vi "EditOptions.vi"(8 "error in":errorcluster, 11 "node in":refnum<class "NISE_CEF_Node.lvclass">) -> (0 "error out":errorcluster, 1 "edit options":T1, 2 "subnodes class":T2, 3 "node out":refnum<class "NISE_CEF_Node.lvclass">)   [LabVIEW 2013, in "NISE_CEF_Node.lvclass"]
doc: "Contains the options for the Menu that will be displayed when doing right click on an item.\nThe sub nodes class configures which nodes can be added to this nodes\nAnd the edit options determine which options are available for the node.\nThis configuration is stored in this VI in case some dynamic configuration is required for the menu options or sub nodes."
uses:
  NISE_CEF_Node.lvclass
  SubNodeCluster.ctl
  NodeMenuOptions.ctl
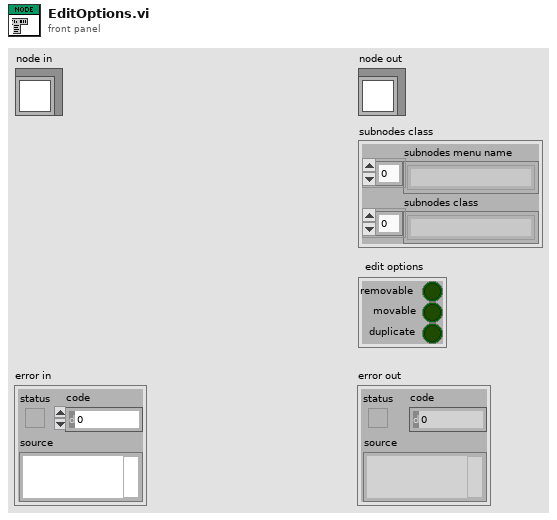
[diagram p1: front panel]
types:
  T1 = typedef "NISE_CEF_Node.lvclass/NodeMenuOptions.ctl" = cluster{"removable":bool, "movable":bool, "duplicate":bool}
  T2 = typedef "NISE_CEF_Node.lvclass/SubNodeCluster.ctl" = cluster{"subnodes menu name":string[], "subnodes class":string[]}
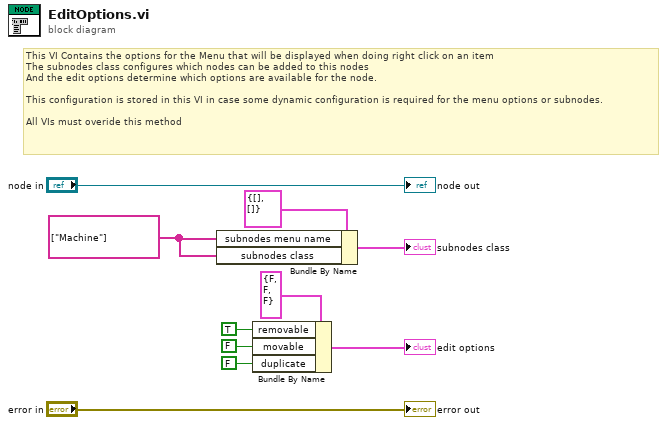
[diagram p0: block diagram]
diagram:
  w2 = string[] ["Machine"] ("subnodes class")
  # "This VI Contains the options for the Menu that will be displayed when doing right click on an item\nThe subnodes class configures which nodes can be added to this nodes\nAnd the edit options determine which options are available for the node.\n\nThis configuration is stored in this VI in case some dynamic configuration is required for the menu options or subnodes.\n\nAll VIs must overide this method"
  n1 = Bundle By Name(cluster=T2 {"subnodes menu name"=[], "subnodes class"=[]} ("subnodes class"), "subnodes menu name"=w2, "subnodes class"=w2) -> (→"subnodes class":T2)
  n2 = Bundle By Name(cluster=T1 {"removable"=FALSE, "movable"=FALSE, "duplicate"=FALSE} ("edit options"), "removable"=TRUE ("Removable"), "movable"=FALSE ("Movable"), "duplicate"=FALSE) -> (→"edit options":T1)
  "error out" <- "error in"
  "node out" <- "node in"
